vi "Set Speed P40.vi"(8 "error in (no error)":errorcluster, 10 "speed (ml/min)":dbl min=0.0 max=999.99 format="%06.2f", 11 "SSI P40 Settings In":T1={"VISA resource name"="", "Simulated?"=TRUE}) -> (0 "error out":errorcluster, 1 "Connection Error":bool, 3 "SSI P40 Settings Out":T1={"VISA resource name"="", "Simulated?"=TRUE})   [LabVIEW 2021, in "SSI P40 Pump.lvlib"]
uses:
  SSI P40 Pump.lvlib
  SSI P40 Settings Cluster.ctl
  SSI PR or LD Pump.lvlib
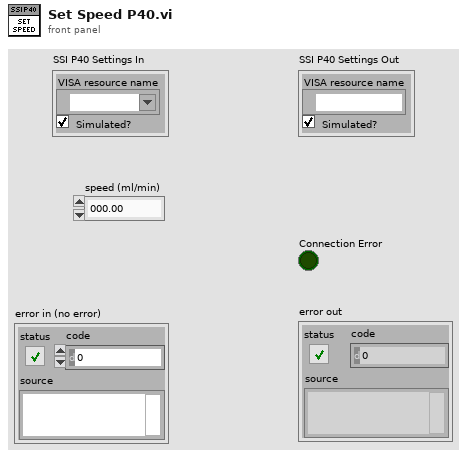
[diagram p1: front panel]
types:
  T1 = typedef "SSI P40 Pump.lvlib/SSI P40 Settings Cluster.ctl" = cluster{"VISA resource name":refnum<visa-resource-name>, "Simulated?":bool}
  T2 = typedef "SSI PR or LD Pump.lvlib/SSI PR or LD Settings Cluster.ctl" = cluster{"VISA resource name":refnum<visa-resource-name>, "Simulated?":bool}
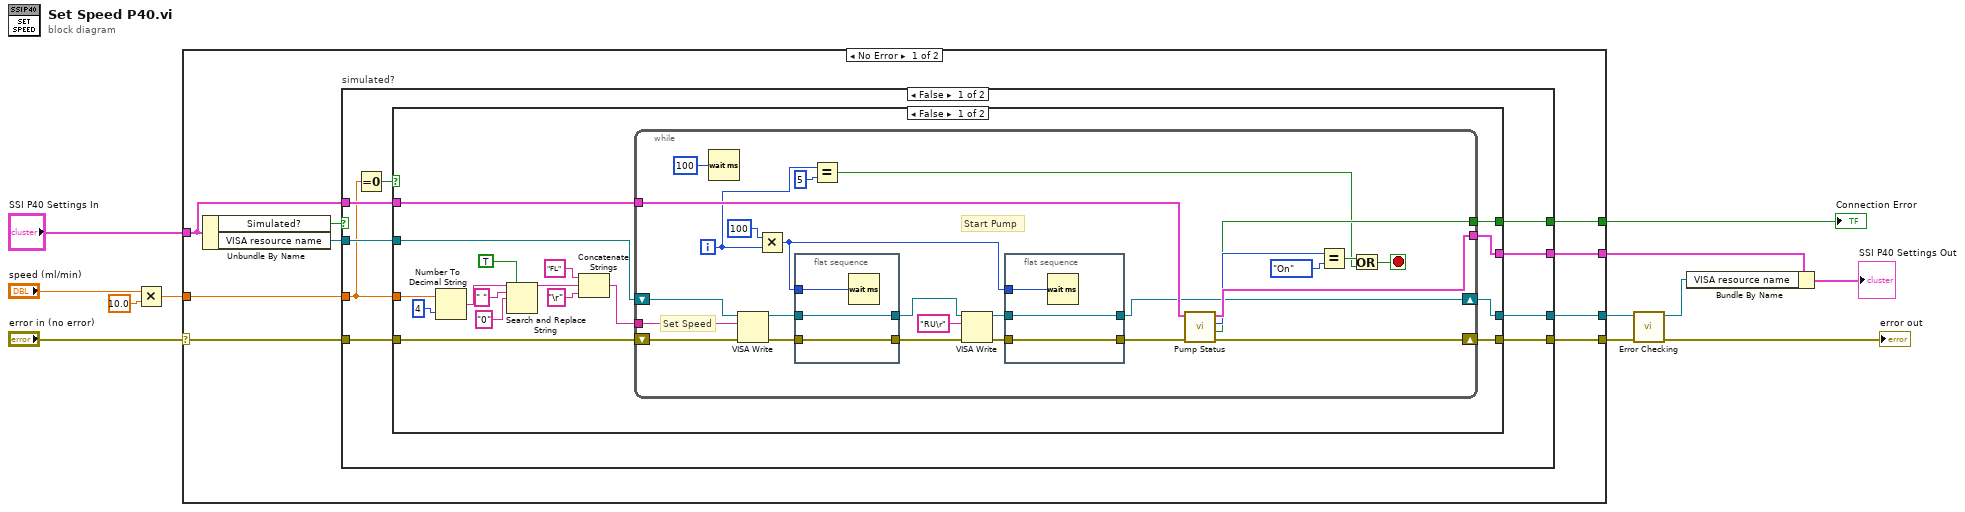
[diagram p0: block diagram]
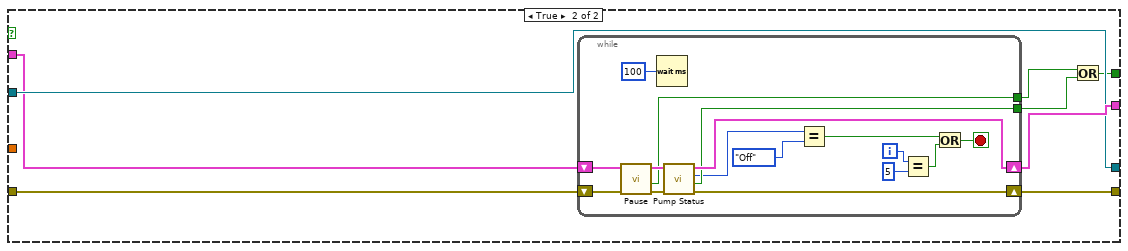
[diagram p2: hidden frame]
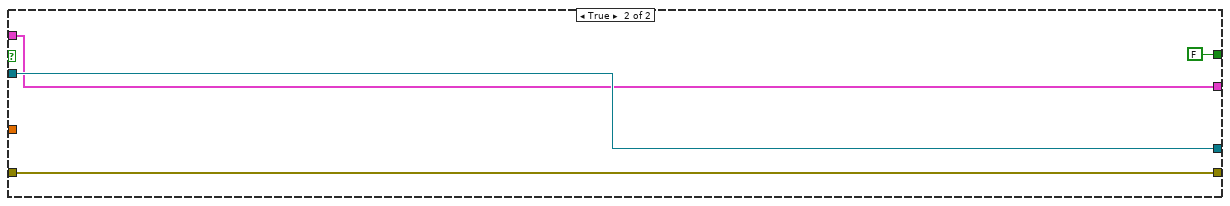
[diagram p3: hidden frame]
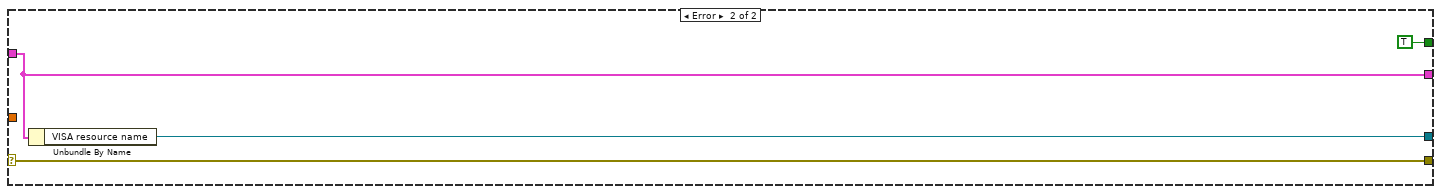
[diagram p4: hidden frame]
diagram:
  n1 = Multiply(x="speed (ml/min)", y=10.0) -> (x*y=w3:dbl)
  n2 = case shown="No Error" "error in (no error)" {
    selector: "error in (no error)" -> [w21 w111]
    tunnel: [w17 w110] -> w8
    tunnel: "SSI P40 Settings In" -> [w18 w110]
    tunnel: [w20 w109] -> w12
    tunnel: [w19 w111] -> w11
    tunnel: [w16 TRUE ("Connection Error")] -> w6
    tunnel: w3 -> [w13 _]
    frame No Error {
      n3 = Unbundle By Name(w18) -> ("Simulated?"=w15:bool, "VISA resource name"=w14:refnum<visa-resource-name>)
      n4 = case "simulated?" shown="False" w15 {
        tunnel: [w28 w107] -> w20
        tunnel: w14 -> [w30 w107]
        tunnel: w21 -> [w29 w106]
        tunnel: [w27 w106] -> w19
        tunnel: w18 -> [w26 w105]
        tunnel: [w25 w105] -> w17
        tunnel: [w24 FALSE ("Connection Error")] -> w16
        tunnel: w13 -> [w22 _]
        frame False {
          n5 = Equal To 0?(x=w22) -> (x = 0?=w23:bool)
          n6 = case shown="False" w23 {
            tunnel: w30 -> [w47 w85]
            tunnel: w29 -> [w46 w83]
            tunnel: [w45 w85] -> w28
            tunnel: [w44 w87] -> w27
            tunnel: w26 -> [w43 w84]
            tunnel: [w42 w86] -> w25
            tunnel: [w41 w80] -> w24
            tunnel: w22 -> [w34 _]
            frame False {
              n7 = Number To Decimal String(number=w34, width (-)=i16 4) -> (decimal integer string=w39:string)
              n8 = Search and Replace String(replace all?=TRUE ("replace all? (F)"), input string=w39, search string=" ", replace string="0" ("replace string (\"\")")) -> (result string=w40:string)  [unwired: 4 in, 3 out]
              n9 = Concatenate Strings("FL" ("string"), w40, "\r" ("string")) -> (w31:string)
              n10 = while {
                shift-right: [w59] -> w45
                shift-left: w47 -> [w66]
                shift-right: [w70] -> w44
                shift-left: w46 -> [w65]
                tunnel: w43 -> [w68]
                tunnel: [w69] -> w42
                tunnel: [w64] -> w41
                tunnel: w31 -> [w48]
                i -> [w51]
                stop <- w52 stop-if-true
                # "Set Speed"
                # "Start Pump"
                n11 = Wait (ms)(milliseconds to wait=u32 100) -> ()  [unwired: 1 out]
                n12 = VISA Write(VISA resource name=w66, write buffer=w48, error in (no error)=w65) -> (VISA resource name out=w62:refnum<visa-resource-name>, error out=w60:errorcluster)  [unwired: 1 out]
                n13 = Multiply(x=u32 100 ("milliseconds to wait"), y=w51) -> (x*y=w49:u32)
                n14 = flat-sequence {
                  tunnel: [w79] -> w63
                  tunnel: w62 -> [w79]
                  tunnel: [w78] -> w61
                  tunnel: w60 -> [w78]
                  tunnel: w49 -> [w77]
                  frame #0 {
                    n15 = Wait (ms)(milliseconds to wait=w77) -> ()  [unwired: 1 out]
                  }
                }
                n16 = Equal?(x=w51, y=5) -> (x = y?=w53:bool)
                n17 = VISA Write(VISA resource name=w63, write buffer="RU\r" ("string"), error in (no error)=w61) -> (VISA resource name out=w58:refnum<visa-resource-name>, error out=w56:errorcluster)  [unwired: 1 out]
                n18 = flat-sequence {
                  tunnel: [w76] -> w59
                  tunnel: w58 -> [w76]
                  tunnel: [w75] -> w57
                  tunnel: w56 -> [w75]
                  tunnel: w49 -> [w74]
                  frame #0 {
                    n19 = Wait (ms)(milliseconds to wait=w74) -> ()  [unwired: 1 out]
                  }
                }
                n20 = call "Pump Status.vi"("error in (no error)"=w57, "SSI PR Settings"=w68) -> ("error out"=w70:errorcluster, "Connection Error"=w64:bool, "Pump On?"=w67:enum16{"Off", "On", "Not Initialized"}, "SSI PR Settings"=w69:T2)  [unwired: 4 in, 2 out]
                n21 = Equal?(x=w67, y=enum16{"Off", "On", "Not Initialized"}."On") -> (x = y?=w54:bool)
                n22 = Or(x=w54, y=w53) -> (x .or. y?=w52:bool)
              }
            }
            frame True {
              n23 = while {
                tunnel: [w97] -> w82
                tunnel: [w96] -> w81
                shift-right: [w102] -> w86
                shift-left: w84 -> [w101]
                shift-right: [w103] -> w87
                shift-left: w83 -> [w100]
                i -> [w89]
                stop <- w90 stop-if-true
                n24 = call "Pause.vi"("error in (no error)"=w100, "SSI PR Settings In"=w101) -> ("error out"=w99:errorcluster, "Connection Error"=w96:bool, "SSI PR Settings Out"=w98:T2)  [unwired: 6 in]
                n25 = Wait (ms)(milliseconds to wait=u32 100) -> ()  [unwired: 1 out]
                n26 = call "Pump Status.vi"("error in (no error)"=w99, "SSI PR Settings"=w98) -> ("error out"=w103:errorcluster, "Connection Error"=w97:bool, "Pump On?"=w92:enum16{"Off", "On", "Not Initialized"}, "SSI PR Settings"=w102:T2)  [unwired: 4 in, 2 out]
                n27 = Equal?(x=w92, y=enum16{"Off", "On", "Not Initialized"}."Off") -> (x = y?=w91:bool)
                n28 = Equal?(x=w89, y=5) -> (x = y?=w93:bool)
                n29 = Or(x=w91, y=w93) -> (x .or. y?=w90:bool)
              }
              n30 = Or(x=w81, y=w82) -> (x .or. y?=w80:bool)
            }
          }
        }
        frame True {
        }
      }
    }
    frame Error {
      n31 = Unbundle By Name(w110) -> ("VISA resource name"=w109:refnum<visa-resource-name>)
    }
  }
  "Connection Error" <- w6
  n32 = call "Error Checking.vi"("error in (no error)"=w11, "VISA resource name"=w12) -> ("error out"=→"error out":errorcluster, "VISA resource name"=w10:refnum<visa-resource-name>)  [unwired: 7 in, 1 out]
  n33 = Bundle By Name(cluster=w8, "VISA resource name"=w10) -> (→"SSI P40 Settings Out":T1)
